vi "Add Status Channels.vi"(8 "error in":errorcluster, 11 "routing and faulting custom device in":T1 format="%.0x") -> (0 "error out":errorcluster, 3 "routing and faulting custom device out":T1 format="%.0x")   [LabVIEW 2020, in "Routing and Faulting Scripting.lvlib"]
uses:
  Routing and Faulting Scripting.lvlib
  <vilib>/NI VeriStand/Custom Device API/Custom Device Item Ref.ctl
  <vilib>/NI VeriStand/Custom Device API/Custom Device Channel.ctl
  <vilib>/NI VeriStand/Custom Device API/Custom Device Channel Type.ctl
  Shared/Constants.vi
  <vilib>/NI VeriStand/Custom Device API/Custom Device API.lvlib
  Shared/Routing and Faulting Shared.lvlib
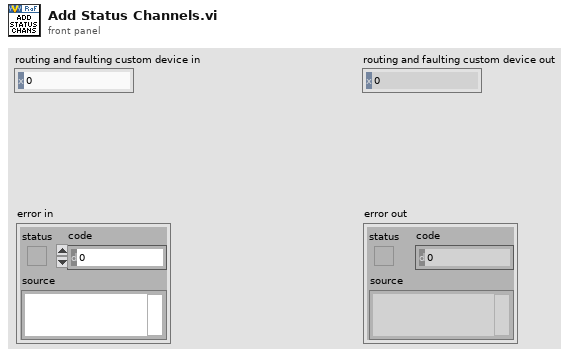
[diagram p1: front panel]
types:
  T1 = typedef "Custom Device API.lvlib/Custom Device Item Ref.ctl" = u64
  T2 = typedef "Custom Device API.lvlib/Custom Device Channel.ctl" = cluster{"Type":T3, "Units":string, "Default Value":dbl, "Faultable":bool, "Scalable":bool}
  T3 = typedef "Custom Device API.lvlib/Custom Device Channel Type.ctl" = enum16{"Input", "Output"}
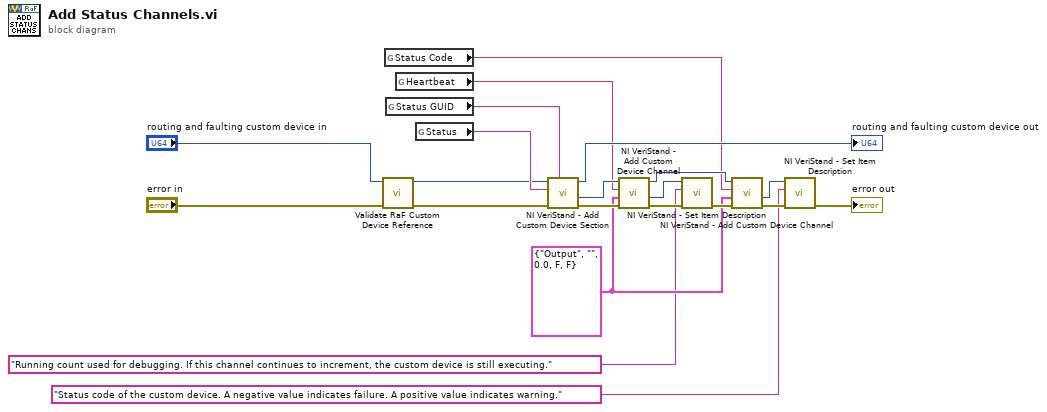
[diagram p0: block diagram]
diagram:
  w8 = T2 {"Type"=enum."Output", "Units"="", "Default Value"=0.0, "Faultable"=FALSE, "Scalable"=FALSE} ("Channel")
  n1 = call "Validate RaF Custom Device Reference.vi"("error in"="error in", "routing and faulting in"="routing and faulting custom device in") -> ("error out"=w3:errorcluster, "routing and faulting out"=w1:T1)  [unwired: 8 in]
  n2 = global read "Constants.vi" "Status Code"() -> (w6:string)
  n3 = global read "Constants.vi" "Status GUID"() -> (w10:string)
  n4 = global read "Constants.vi" "Heartbeat"() -> (w7:string)
  n5 = global read "Constants.vi" "Status"() -> (w9:string)
  n6 = call <vilib>:"NI VeriStand - Add Custom Device Section.vi"("GUID (Default Section)"=w10, "error in (no error)"=w3, "Section Name"=w9, "Parent Ref in"=w1) -> ("error out"=w21:errorcluster, "Section Ptr"=w20:T1, "Parent Ref out"=→"routing and faulting custom device out":T1)  [unwired: 4 in, 1 out]
  n7 = call <vilib>:"NI VeriStand - Add Custom Device Channel.vi"("error in (no error)"=w21, "Channel"=w8, "Channel Name"=w7, "Parent Ref in"=w20) -> ("error out"=w19:errorcluster, "Channel Ref"=w18:T1, "Parent Ref out"=w16:T1)  [unwired: 4 in, 1 out]
  n8 = call <vilib>:"NI VeriStand - Set Item Description.vi"("error in (no error)"=w19, "Description"="Running count used for debugging. If this channel continues to increment, the custom device is still executing.", "Item Ref in"=w18) -> ("error out"=w17:errorcluster)  [unwired: 6 in, 2 out]
  n9 = call <vilib>:"NI VeriStand - Add Custom Device Channel.vi"("error in (no error)"=w17, "Channel"=w8, "Channel Name"=w6, "Parent Ref in"=w16) -> ("error out"=w15:errorcluster, "Channel Ref"=w14:T1)  [unwired: 4 in, 2 out]
  n10 = call <vilib>:"NI VeriStand - Set Item Description.vi"("error in (no error)"=w15, "Description"="Status code of the custom device. A negative value indicates failure. A positive value indicates warning.", "Item Ref in"=w14) -> ("error out"=→"error out":errorcluster)  [unwired: 6 in, 2 out]
